vi "Promise Chain Polling Example.vi"() -> ()   [LabVIEW 2020, in "Futures-Examples.lvlib"]
uses:
  Futures-Examples.lvlib
  DoubleValue/DoubleValue.lvclass/DoubleValue.ctl
  Promises/Promise/Promise.lvclass/Promise.ctl
  Promises/Future/Future.lvclass/Future.ctl
  StringValue/StringValue.lvclass
  C:/dev/lv/2020/lv-promises/Promises/Value/Value.lvclass
  StringValue/StringValue.lvclass/StringValue.ctl
  c8732dd6-9988-450c-b28a-380696434648.vi
  6faf1596-12c2-41e2-be15-7c399fc9a4c1.vi
  bb59f894-ea3b-4805-9a30-f725ab95dd66.vi
  0578e0a0-3799-4f3a-a9f7-df31b47d9f36.vi
  DoubleValue/DoubleValue.lvclass
  Promises/Future/Future.lvclass
  Promises/Promise/Promise.lvclass
panel:
  out "Poll Time mS":u32(graph)
  out "Final Wait mS":i32
  out "error out":errorcluster
  out "Value":string
  out "Loop Count":i32
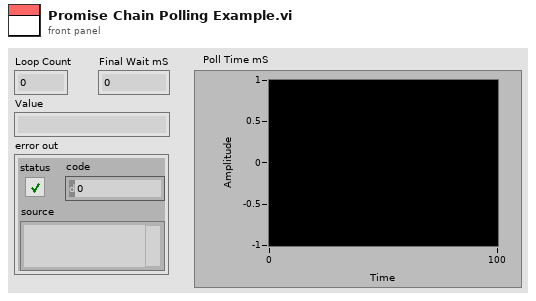
[diagram p1: front panel]
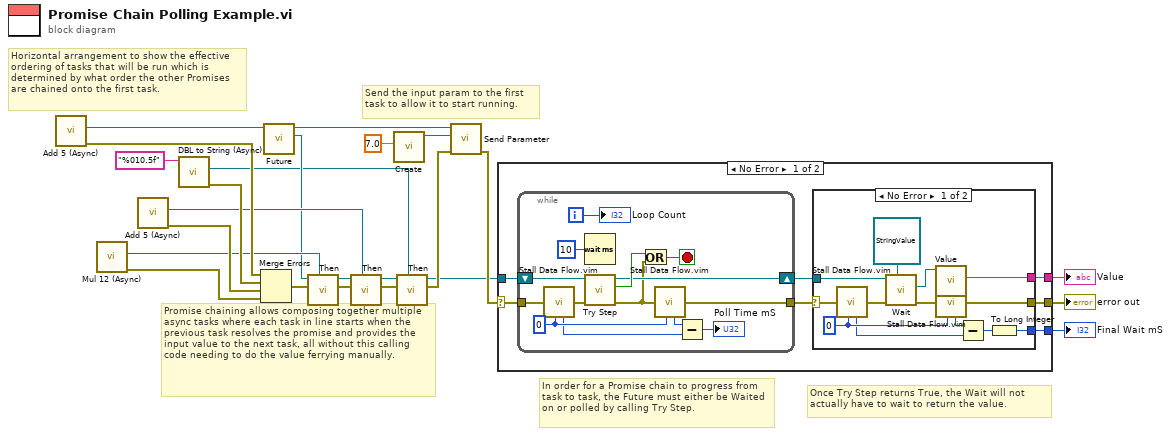
[diagram p0: block diagram]
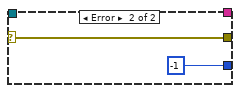
[diagram p2: hidden frame]
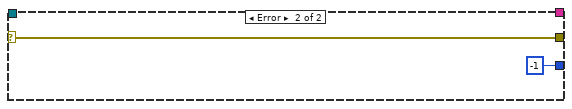
[diagram p3: hidden frame]
diagram:
  # "Horizontal arrangement to show the effective ordering of tasks that will be run which is determined by what order the other Promises are chained onto the first task."
  # "Send the input param to the first task to allow it to start running."
  # "Promise chaining allows composing together multiple async tasks where each task in line starts when the previous task resolves the promise and provides the input value to the next task, all without this calling code needing to do the value ferrying manually."
  # "Once Try Step returns True, the Wait will not actually have to wait to return the value."
  # "In order for a Promise chain to progress from task to task, the Future must either be Waited on or polled by calling Try Step."
  n1 = call "Add 5 (Async).vi"() -> ("error out"=w24:errorcluster, "Add 5 Promise"=w21:refnum<class "Promise.lvclass">)  [unwired: 10 in]
  n2 = call "Mul 12 (Async).vi"() -> ("error out"=w3:errorcluster, "Mul 12 Promise"=w20:refnum<class "Promise.lvclass">)  [unwired: 10 in]
  n3 = call "Add 5 (Async).vi"() -> ("error out"=w22:errorcluster, "Add 5 Promise"=w18:refnum<class "Promise.lvclass">)  [unwired: 10 in]
  n4 = call "DBL to String (Async).vi"("Format String"="%010.5f") -> ("error out"=w23:errorcluster, "Promise out"=w1:refnum<class "Promise.lvclass">)  [unwired: 9 in]
  n5 = Merge Errors(w24, w23, w22, w3) -> (w14:errorcluster)
  n6 = call "Future.vi"("Promise in"=w21) -> ("Future"=w13:refnum<class "Future.lvclass">, "Promise"=w17:refnum<class "Promise.lvclass">)  [unwired: 9 in]
  n7 = call "Then.vi"("Then Promise"=w20, "error in (no error)"=w14, "Future in"=w13) -> ("error out"=w15:errorcluster, "Future out"=w19:refnum<class "Future.lvclass">)  [unwired: 7 in]
  n8 = call "Then.vi"("Then Promise"=w18, "error in (no error)"=w15, "Future in"=w19) -> ("error out"=w11:errorcluster, "Future out"=w12:refnum<class "Future.lvclass">)  [unwired: 7 in]
  n9 = call "Create.vi"("Value"=7.0) -> ("DoubleValue"=w8:refnum<class "DoubleValue.lvclass">)  [unwired: 10 in]
  n10 = call "Then.vi"("Then Promise"=w1, "error in (no error)"=w11, "Future in"=w12) -> ("error out"=w9:errorcluster, "Future out"=w6:refnum<class "Future.lvclass">)  [unwired: 7 in]
  n11 = call "Send Parameter.vi"("error in (no error)"=w9, "Parameter"=w8, "Promise in"=w17) -> ("error out"=w7:errorcluster)  [unwired: 7 in, 1 out]
  n12 = case shown="No Error" w7 {
    selector: w7 -> [w26 w62]
    tunnel: w6 -> [w31 _]
    tunnel: [w28 _] -> w5
    tunnel: [w27 w62] -> w4
    tunnel: [w25 -1] -> w2
    frame No Error {
      n13 = while {
        shift-right: [w57] -> w29
        shift-left: w31 -> [w60]
        tunnel: [w51] -> w30
        tunnel: w26 -> [w53]
        i -> [w56]
        stop <- w58 stop-if-true
        w50 = u32 0 ("milliseconds to wait")
        n14 = call "Stall Data Flow.vim"("value in"=w53, "milliseconds to wait"=w50) -> ("millisecond timer value"=w48:u32, "value out"=w54:errorcluster)
        n15 = Wait (ms)(milliseconds to wait=u32 10) -> ()  [unwired: 1 out]
        n16 = call "Try Step.vi"("error in (no error)"=w54, "Future in"=w60) -> ("error out"=w52:errorcluster, "Ready"=w59:bool, "Future out"=w57:refnum<class "Future.lvclass">)  [unwired: 7 in]
        n17 = Or(x=w59, y=w52) -> (x .or. y?=w58:bool)
        n18 = call "Stall Data Flow.vim"("value in"=w52, "milliseconds to wait"=w50) -> ("millisecond timer value"=w49:u32, "value out"=w51:errorcluster)
        n19 = Subtract(x=w49, y=w48) -> (x-y=→"Poll Time mS":u32)
        "Loop Count" <- w56
      }
      n20 = case shown="No Error" w30 {
        selector: w30 -> [w43 w46]
        tunnel: w29 -> [w44 _]
        tunnel: [w40 _] -> w28
        tunnel: [w36 w46] -> w27
        tunnel: [w32 -1] -> w25
        frame No Error {
          w37 = u32 0 ("milliseconds to wait")
          n21 = call "Stall Data Flow.vim"("value in"=w43, "milliseconds to wait"=w37) -> ("millisecond timer value"=w34:u32, "value out"=w39:errorcluster)
          n22 = call "Wait.vi"("Result Type"=refnum<class "StringValue.lvclass"> refnum ("Futures-Examples.lvlib:StringValue.lvclass"), "error in (no error)"=w39, "Future in"=w44) -> ("error out"=w38:errorcluster, "Result"=w41:refnum<class "StringValue.lvclass">)  [unwired: 7 in]
          n23 = call "Value.vi"("StringValue in"=w41) -> ("Value"=w40:string)  [unwired: 10 in]
          n24 = call "Stall Data Flow.vim"("value in"=w38, "milliseconds to wait"=w37) -> ("millisecond timer value"=w35:u32, "value out"=w36:errorcluster)
          n25 = Subtract(x=w35, y=w34) -> (x-y=w33:u32)
          n26 = To Long Integer(number=w33) -> (32bit integer=w32:i32)
        }
        frame Error {
        }
      }
    }
    frame Error {
    }
  }
  "Value" <- w5
  "error out" <- w4
  "Final Wait mS" <- w2
